vi "Example 7 - Remapping Tags.vi"() -> ()   [LabVIEW 2021]
uses:
  Omni-Bus/Omni_Bus.lvclass
  Omni-Bus/Support/Broad Types.ctl
  Local Bus/Local Bus.lvclass
  C:/Users/Tim/Documents/GitHub/Omni-Bus/Source/Omni-Bus/Bus Access/Bus_Access.lvclass
  <vilib>/Utility/Data Type/Type Definitions/Data Type.ctl
  Remap Bus/Remap Bus.lvclass
  Aggregator Bus/Aggregator Bus.lvclass
  Omni-Bus/Support/Write/Write DBL.vi
  Omni-Bus/Support/Read/Read DBL.vi
  <vilib>/TSA/Abstract Data Classes/Constants/Support/DBL/Const_DBL.lvclass
  C:/Program Files (x86)/National Instruments/LabVIEW 2021/vi.lib/TSA/Abstract Data Classes/Abs_Types/Type/Abs_Type.lvclass
  <vilib>/TSA/Abstract Data Classes/Constants/Support/DBL/DBL.vi
  <vilib>/TSA/Abstract Data Classes/Abs_Types/Double Float/Abs_Double Float.lvclass
  <vilib>/Utility/Data Type/NI_Data Type.lvlib
panel:
  in  "Keep Original Tag":bool
  out "Numeric 4":dbl
  out "Numeric 3":dbl
  in  "Numeric 2":dbl
  in  "Numeric":dbl
  in  "Write DBL Tag":string(combo)
  out "Write DBL error":errorcluster
  in  "Write DBL Tag":string(combo)
  out "Write DBL error":errorcluster
  out "Read DBL Error":errorcluster
  out "Read DBL error":errorcluster
  in  "Read DBL Tag":string(combo)
  in  "Read DBL Tag":string(combo)
  out "Read DBL error":errorcluster
  out "Write DBL error":errorcluster
  in  "Double":dbl
  in  "Write DBL Tag":string(combo)
  in  "stop":bool
  out "Double":dbl format="%.2f"
  in  "Read DBL Tag":string(combo)
  out "error out":errorcluster
  out "All Tags":string[](array[string])
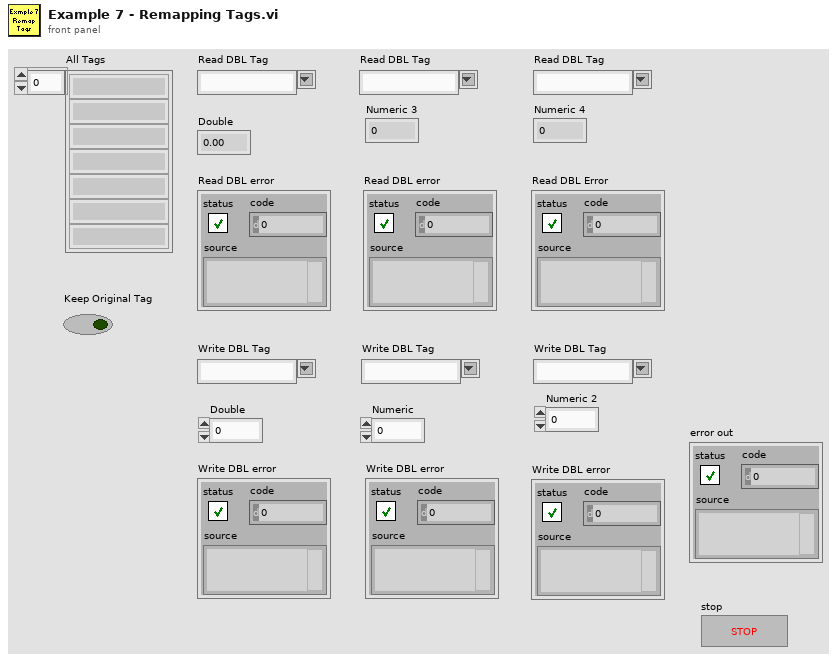
[diagram p1: front panel]
types:
  T1 = typedef "NI_Data Type.lvlib/Data Type.ctl" = enum8{"Invalid Type", "Void", "I8", "I16", "I32", "I64", "U8", "U16", "U32", "U64", "Single Float", "Double Float", "Extended Float", "Single Complex", "Double Complex", "Extended Complex", "Enum U8", "Enum U16", "Enum U32", "Enum U64", "Single Float With Unit", "Double Float With Unit", "Extended Float With Unit", "Single Complex with Unit", "Double Complex with Unit", "Extended Complex with Unit", "Boolean", "String", "Path", "Picture", "Tag", "Array", "Cluster", "Variant", "LV Variant", "Waveform", "Timestamp", "Digital Waveform", "Digital Data", "ExpressData", "Refnum", "External Data", "VI", "Poly VI", "LabVIEW Class Instance", "Fixed Point", "Set Collection", "Map Collection"}
  T2 = typedef "Omni_Bus.lvclass/Broad Types.ctl" = enum16{"All Tags", "NI Specific Type", "Boolean", "String", "Numeric", "Float", "Integer", "Collection", "All Value Types", "Non Value Types"}
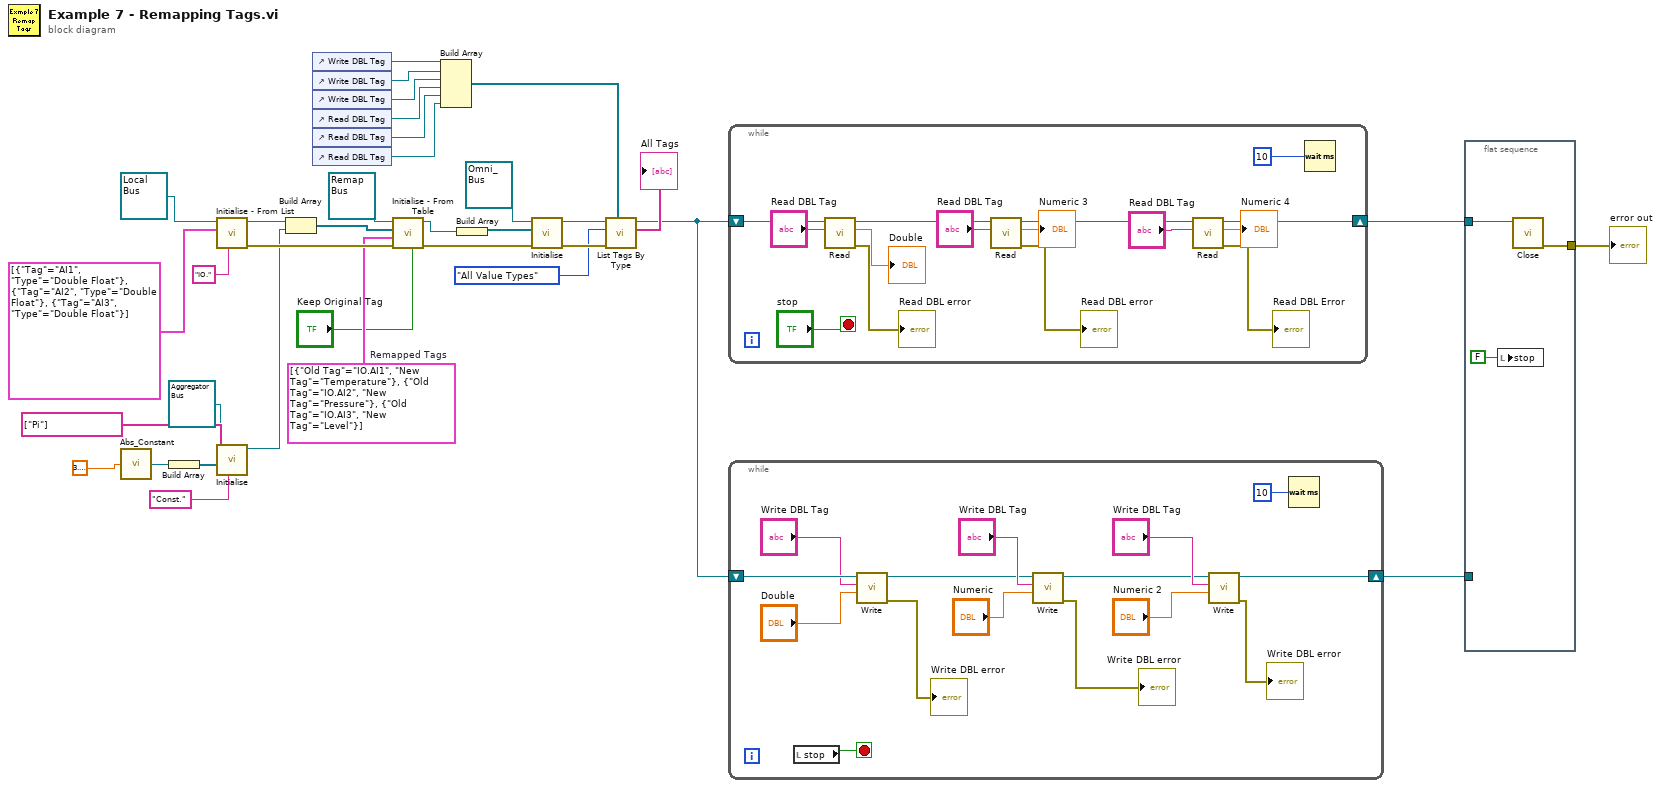
[diagram p0: block diagram]
diagram:
  w21 = cluster{"Old Tag":string, "New Tag":string}[] [{"Old Tag"="IO.AI1", "New Tag"="Temperature"}, {"Old Tag"="IO.AI2", "New Tag"="Pressure"}, {"Old Tag"="IO.AI3", "New Tag"="Level"}]  # Remapped Tags
  n1 = call-poly <vilib>:"Abs_Constant.vi"("Value"=3.141592653589793) -> ("Constant"=w17:refnum<class "Const_DBL.lvclass">)  [unwired: 4 in]
  n2 = Build Array(w17) -> (w18:refnum<class "Const_DBL.lvclass">[])
  n3 = call "Initialise - From List.vi"("Tag Root"="IO.", "Tag List"=cluster{"Tag":string, "Type":T1}[] [{"Tag"="AI1", "Type"=enum."Double Float"}, {"Tag"="AI2", "Type"=enum."Double Float"}, {"Tag"="AI3", "Type"=enum."Double Float"}], "Local Bus in"=refnum<class "Local Bus.lvclass"> refnum ("Local Bus.lvclass")) -> ("error out"=w22:errorcluster, "Local Bus out"=w26:refnum<class "Local Bus.lvclass">)  [unwired: 7 in]
  n4 = call "Initialise.vi"("Tag Root"="Const.", "Values"=w18, "Tags"=string[] ["Pi"], "Aggregator Bus in"=refnum<class "Aggregator Bus.lvclass"> refnum) -> ("Aggregator Bus out"=w19:refnum<class "Aggregator Bus.lvclass">)  [unwired: 6 in, 1 out]
  n5 = Build Array(w26, w19) -> (w23:refnum<class "Bus_Access.lvclass">[])
  n6 = control-ref of="Write DBL Tag"() -> (w10:refnum<vi>)
  n7 = control-ref of="Write DBL Tag"() -> (w9:refnum<vi>)
  n8 = control-ref of="Write DBL Tag"() -> (w8:refnum<vi>)
  n9 = control-ref of="Read DBL Tag"() -> (w7:refnum<vi>)
  n10 = control-ref of="Read DBL Tag"() -> (w6:refnum<vi>)
  n11 = control-ref of="Read DBL Tag"() -> (w5:refnum<vi>)
  n12 = call "Initialise - From Table.vi"("Keep Original Tag"="Keep Original Tag", "error in (no error)"=w22, "Remapped Tags"=w21, "Buses"=w23, "Remap Bus in"=refnum<class "Remap Bus.lvclass"> refnum) -> ("error out"=w20:errorcluster, "Remap Bus out"=w14:refnum<class "Remap Bus.lvclass">)  [unwired: 5 in]
  n13 = Build Array(w10, w9, w8, w7, w6, w5) -> (w4:refnum<vi>[])
  n14 = Build Array(w14) -> (w13:refnum<class "Remap Bus.lvclass">[])
  n15 = call-dynamic "Initialise.vi"("error in (no error)"=w20, "Bus Access"=w13, "Var Bus in"=refnum<class "Omni_Bus.lvclass"> refnum) -> ("error out"=w33:errorcluster, "Var Bus out"=w34:refnum<class "Omni_Bus.lvclass">)  [unwired: 7 in]
  n16 = call-dynamic "List Tags By Type.vi"("Combo Boxes"=w4, "error in (no error)"=w33, "Broad Types"=Broad_Types."All Value Types", "Var Bus in"=w34) -> ("Tags"=→"All Tags":string[], "Var Bus out"=w28:refnum<class "Omni_Bus.lvclass">)  [unwired: 4 in, 2 out]
  n17 = while {
    shift-right: [w40] -> w29
    shift-left: w28 -> [w50]
    stop <- "stop" stop-if-true
    n18 = call-poly "Read.vi"("Tag"="Read DBL Tag", "Var Bus in"=w50) -> ("error out"=→"Read DBL error":errorcluster, "Numeric"=→"Double":dbl, "Var Bus out"=w43:refnum<class "Omni_Bus.lvclass">)  [unwired: 7 in]
    n19 = call-poly "Read.vi"("Tag"="Read DBL Tag", "Var Bus in"=w43) -> ("error out"=→"Read DBL error":errorcluster, "Numeric"=→"Numeric 3":dbl, "Var Bus out"=w41:refnum<class "Omni_Bus.lvclass">)  [unwired: 7 in]
    n20 = call-poly "Read.vi"("Tag"="Read DBL Tag", "Var Bus in"=w41) -> ("error out"=→"Read DBL Error":errorcluster, "Numeric"=→"Numeric 4":dbl, "Var Bus out"=w40:refnum<class "Omni_Bus.lvclass">)  [unwired: 7 in]
    n21 = Wait (ms)(milliseconds to wait=u32 10) -> ()  [unwired: 1 out]
  }
  n22 = while {
    shift-right: [w53] -> w27
    shift-left: w28 -> [w65]
    stop <- w62 stop-if-true
    n23 = local read "stop"() -> (w62:bool)
    n24 = call-poly "Write.vi"("Numeric"="Double", "Tag"="Write DBL Tag", "Omni_Bus in"=w65) -> ("error out"=→"Write DBL error":errorcluster, "Omni_Bus out"=w57:refnum<class "Omni_Bus.lvclass">)  [unwired: 7 in]
    n25 = call-poly "Write.vi"("Numeric"="Numeric", "Tag"="Write DBL Tag", "Omni_Bus in"=w57) -> ("error out"=→"Write DBL error":errorcluster, "Omni_Bus out"=w54:refnum<class "Omni_Bus.lvclass">)  [unwired: 7 in]
    n26 = call-poly "Write.vi"("Numeric"="Numeric 2", "Tag"="Write DBL Tag", "Omni_Bus in"=w54) -> ("error out"=→"Write DBL error":errorcluster, "Omni_Bus out"=w53:refnum<class "Omni_Bus.lvclass">)  [unwired: 7 in]
    n27 = Wait (ms)(milliseconds to wait=u32 10) -> ()  [unwired: 1 out]
  }
  n28 = flat-sequence {
    tunnel: [w68] -> w30
    tunnel: w29 -> [w67]
    tunnel: w27 -> [_]
    frame #0 {
      n29 = local write "stop"(FALSE ("stop")) -> ()
      n30 = call-dynamic "Close.vi"("Data in"=w67) -> ("error out"=w68:errorcluster)  [unwired: 9 in, 1 out]
    }
  }
  "error out" <- w30
